vi "Test Increment File Name.vi"(8 "error in (no error)":errorcluster, 11 "LVtoITX in":refnum<class "LVtoITX.lvclass">) -> (0 "error out":errorcluster, 3 "LVtoITX out":refnum<class "LVtoITX.lvclass">)   [LabVIEW 2016, in "LVtoITX.lvclass"]
uses:
  LVtoITX.lvclass
panel:
  in  "stop":bool=TRUE
  out "XY Graph":cluster{i32[], u32[]}(graph)
  out "Numeric":i32=5699
  out "x-y":u32=5
  in  "path":path=path "C:/user/patrick/other/test/filename.itx"
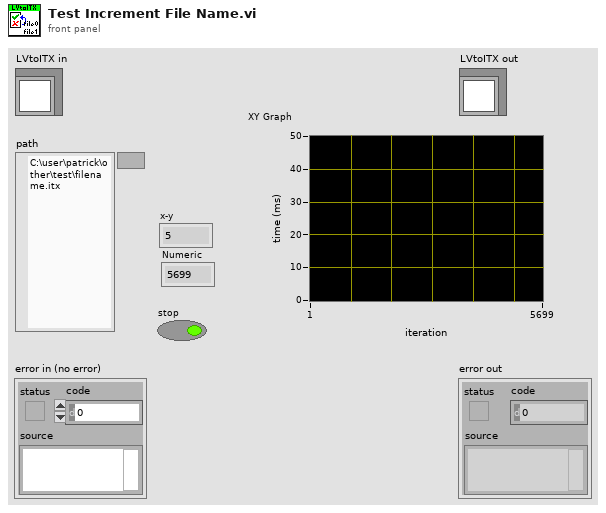
[diagram p1: front panel]
types:
  T1 = enum16{"open", "replace", "create", "open or create", "replace or create", "replace or create with confirmation"}
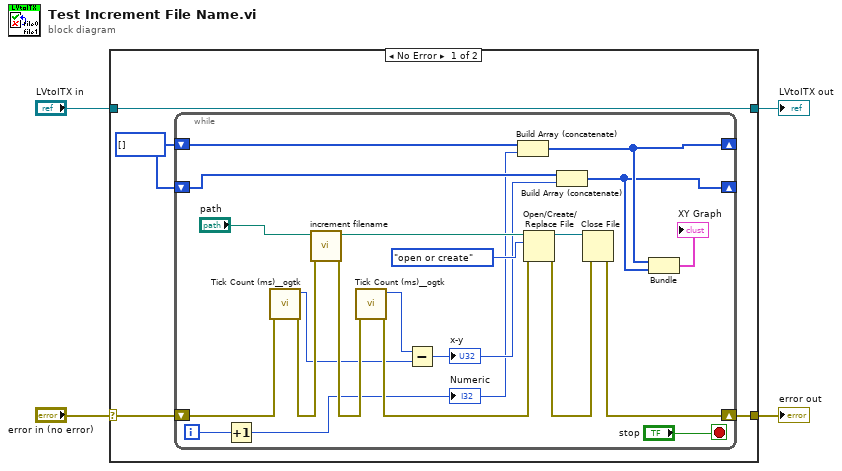
[diagram p0: block diagram]
diagram:
  n1 = case shown="No Error" "error in (no error)" {
    selector: "error in (no error)" -> [w7 w31]
    tunnel: [w6 w31] -> w3
    tunnel: [w8 w30] -> w1
    tunnel: "LVtoITX in" -> [w8 w30]
    frame No Error {
      w5 = i32[] []
      n2 = while {
        shift-right: [w25] -> w6
        shift-left: w7 -> [w23]
        shift-right: [w12] -> _
        shift-left: w5 -> [w14]
        shift-right: [w11] -> _
        shift-left: w5 -> [w13]
        i -> [w16]
        stop <- "stop" stop-if-true
        n3 = Increment(x=w16) -> (x+1=w9:i32)
        "Numeric" <- w9
        n4 = call <userlib>:"Tick Count (ms)__ogtk.vi"("error in (no error)"=w23) -> ("error out"=w24:errorcluster, "millisecond timer value"=w19:u32)  [unwired: 9 in]
        n5 = call <userlib>:"increment filename.vi"("error in (no error)"=w24, "path"="path") -> ("error out"=w22:errorcluster, "modified path"=w28:path)  [unwired: 8 in]
        n6 = call <userlib>:"Tick Count (ms)__ogtk.vi"("error in (no error)"=w22) -> ("error out"=w21:errorcluster, "millisecond timer value"=w20:u32)  [unwired: 9 in]
        n7 = Subtract(x=w20, y=w19) -> (x-y=w15:u32)
        "x-y" <- w15
        n8 = Build Array (concatenate)(w14, w9) -> (w12:i32[])
        n9 = Open/Create/Replace File(file path (use dialog)=w28, error in=w21, operation (0:open)=T1."open or create") -> (refnum out=w26:refnum<file>, error out=w27:errorcluster)  [unwired: 3 in, 1 out]
        n10 = Build Array (concatenate)(w13, w15) -> (w11:u32[])
        n11 = Close File(refnum=w26, error in=w27) -> (error out=w25:errorcluster)  [unwired: 1 out]
        n12 = Bundle(w12, w11) -> (→"XY Graph":cluster{i32[], u32[]})  [unwired: 1 in]
      }
    }
    frame Error {
    }
  }
  "error out" <- w3
  "LVtoITX out" <- w1
